vi "Save_Info.vi"(8 "error in (no error)":errorcluster, 11 "AB_WebService in":refnum<class "AB_WebService.lvclass">) -> (0 "error out":errorcluster, 3 "AB_WebService out":refnum<class "AB_WebService.lvclass">)   [LabVIEW 2020, in "AB_WebService.lvclass"]
uses:
  <vilib>/AppBuilder/AB_Classes/WebService/AB_WebService.lvclass
  e:/builds/penguin/labview/branches/2020/dev/dist/vi.lib/AppBuilder/AB_Classes/Build/AB_Build.lvclass
  <vilib>/Utility/error.llb/whitespace.ctl
  <vilib>/AppBuilder/RW_Project/AB_RW_Project_WebService_Data.ctl
  <vilib>/AppBuilder/RW_Project/AB_RW_Project_PropBag_Action.ctl
  <vilib>/AppBuilder/AB_Classes/WebService/AB_WebService.lvclass/AB_WebService.ctl
  <vilib>/AppBuilder/AB_Classes/TargetFile/AB_Targetfile.lvclass
  <vilib>/AppBuilder/AB_Classes/Build/AB_Build.lvclass
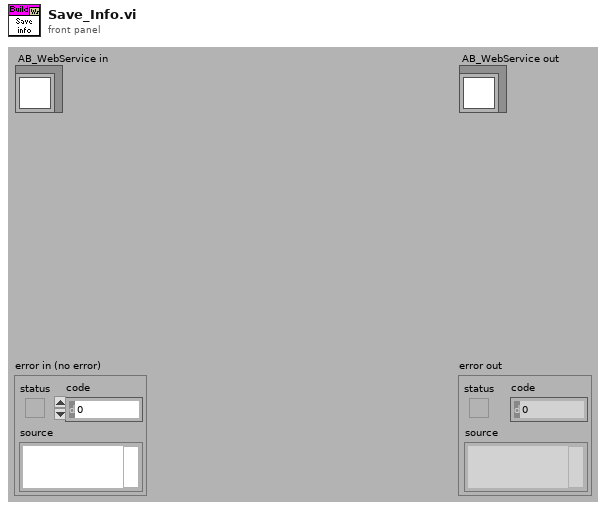
[diagram p1: front panel]
types:
  T1 = typedef "whitespace.ctl" = u16
  T2 = typedef "AB_RW_Project_WebService_Data.ctl" = cluster{"service aliases":string, "standalone":bool}
  T3 = typedef "AB_RW_Project_PropBag_Action.ctl" = enum16{"read", "write", "clear", "readPrevious", "writePrevious", "clearPrevious"}
  T4 = typedef "AB_WebService.ctl" = cluster{"service aliases":string[], "standalone":bool}
  T5 = typedef "AB_Build.ctl" = cluster{"buildSpecName":string, "buildSpecDescription":string, "destinations":refnum<class "AB_Destination.lvclass">[], "exclusionOption":T6, "defaultLanguage":string, "supportedLanguages":string[], "excludedDirectories":path[], "buildContext":refnum<vi>, "buildObject":T7, "preview":bool, "programatic":bool, "progressBarEvents":T8, "userLog_Path":path, "preActionID":string, "preAction_Path":path, "postActionID":string, "postAction_Path":path, "eng_checkForBrokenVIs?":bool, "eng_verboseLinkerErrors?":bool, "localDest_Path":path, "targetDest_Path":path, "removeVIObject":u16, "cache":refnum<class "PreviewCache.lvclass">, "use cache":bool, "previewCache_ID":string, "buildCache_ID":string, "eng_TempLocalDest_Path":path, "eng_collectDependencies?":bool, "versionInfo":cluster{"buildVersion":cluster{"major":u16, "minor":u16, "patch":u16, "build":u16}, "autoIncrement":bool}, "eng_enableVIChecksums":bool}
  T6 = typedef "AB_Exclusion_Option.ctl" = cluster{"typedefs":bool, "polymorphicVIs":bool, "unusedLibraryItems":bool, "modifyLibraryFile":bool, "edit-timeDependencies":bool, "inlineVIs":bool, "dependent PPLs":bool, "dependent DLLs":bool}
  T7 = typedef "ItemRef.ctl" = u64
  T8 = typedef "provcom_ProgressBar_Events.ctl" = cluster{"newJob":refnum<user-event>, "newItem":refnum<user-event>, "errorMsg":T9, "cancel":refnum<user-event>}
  T9 = typedef "mxLvBuildError.ctl" = refnum<user-event>
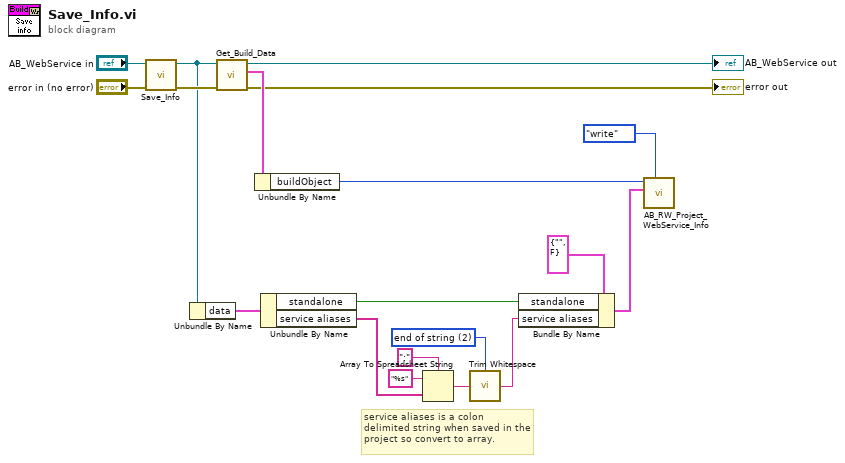
[diagram p0: block diagram]
diagram:
  w4 = T1 2 items=["both", "start of string", "end of string"] ("location (both)")
  # "service aliases is a colon delimited string when saved in the project so convert to array."
  n1 = call-parent "Save_Info.vi"("error in (no error)"="error in (no error)", "AB_Targetfile in"="AB_WebService in") -> ("error out"=w15:errorcluster, "AB_Targetfile out"=w13:refnum<class "AB_WebService.lvclass">)  [unwired: 8 out]
  n2 = Unbundle By Name(w13) -> ("data"=w9:T4)
  n3 = call <vilib>:"Get_Build_Data.vi"("error in (no error)"=w15, "Class in"=w13) -> ("error out"=→"error out":errorcluster, "data"=w17:T5, "Class out"=→"AB_WebService out":refnum<class "AB_WebService.lvclass">)  [unwired: 7 out]
  n4 = Unbundle By Name(w17) -> ("buildObject"=w1:T7)
  n5 = Unbundle By Name(w9) -> ("standalone"=w2:bool, "service aliases"=w6:string[])
  n6 = Array To Spreadsheet String(delimiter (Tab)=":", array=w6, 3:"%s" ("format string")) -> (spreadsheet string=w5:string)
  n7 = call <vilib>:"Trim Whitespace.vi"("string"=w5, "location (both)"=w4) -> ("trimmed string"=w3:string)
  n8 = Bundle By Name(cluster=T2 {"service aliases"="", "standalone"=FALSE} ("webServiceInfo in"), "standalone"=w2, "service aliases"=w3) -> (w10:T2)
  n9 = call <vilib>:"AB_RW_Project_WebService_Info.vi"("action"=AB_RW_Project_PropBag_Action."write", "webServiceInfo in"=w10, "Object In"=w1) -> ()  [unwired: 1 in, 8 out]
